vi "Prototype with Standard Deviation.vi"() -> ()   [LabVIEW 2012]
doc: "Use this template to build a standard state machine design pattern. Each state executes code and determines which state to transition to. Contrast this design pattern with the User Interface Event Handler pattern, in which code executes in response to user actions. Contrast this design pattern also with the Queued Message Handler pattern, in which each message handling code can queue zero or more new messages.\nNote: This template does not contain the most recent programming guidelines recommended by National Instruments. For a complete, project-based implementation of the Standard State Machine pattern, use the Create Project dialog box instead of this template."
uses:
  <vilib>/Math Plots/3D Math Plots/3D Bar/3D Bar Datatype/3D Bar Datatype.lvclass
  <vilib>/Math Plots/3D Math Plots/3D Bar/3D Bar Datatype/Public/Plot Helper (Vector).vi
  <vilib>/Math Plots/3D Math Plots/3D Bar/3D Bar XCtrl/3D Bar.xctl
panel:
  out "Tramp contact":bool
  out "3D Bar Graph":refnum<class "3D Plot Datatype.lvclass">[](xcontrol)
  out "Total Air Time":dbl
  out "Number of\nTotal Jumps":i32
  out "Number of Official Jumps":i32
  in  "Start Official Jumps \n(Represents Current State)":bool
  out "Final Jump Times":dbl[](array[numeric])
  out "Trampoline Time":dbl[](array[numeric])
  out "Air Time":dbl[](array[numeric])
  in  "Stop":bool
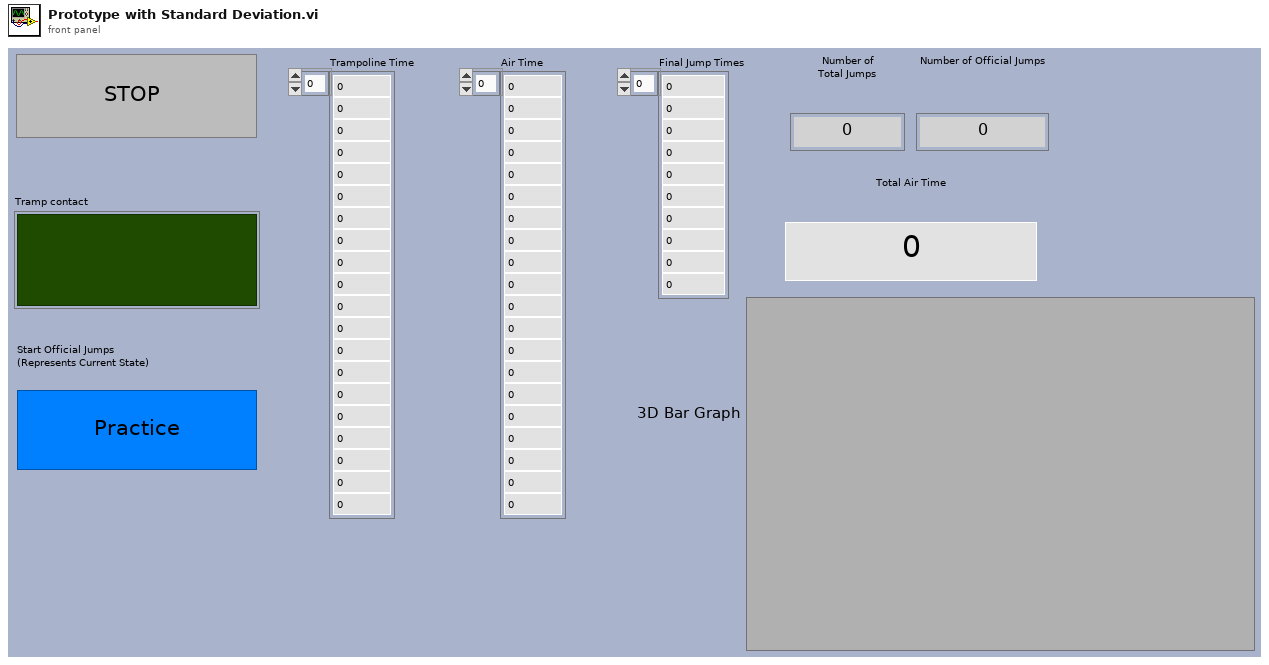
[diagram p1: front panel]
types:
  T1 = cluster{"On Trampoline":bool, "Timestamp":timestamp}
  T2 = cluster{"Start Time":dbl, "Air Time Array ":dbl[], "Tramp Time Array":dbl[], "Number of Jumps  ":i32, "Tramp switch":bool, "Final Time Array":dbl[], "Number of Final Jumps":i32}
  T3 = enum16{"Initialize", "acquire", "analyze", "display", "Stop"}
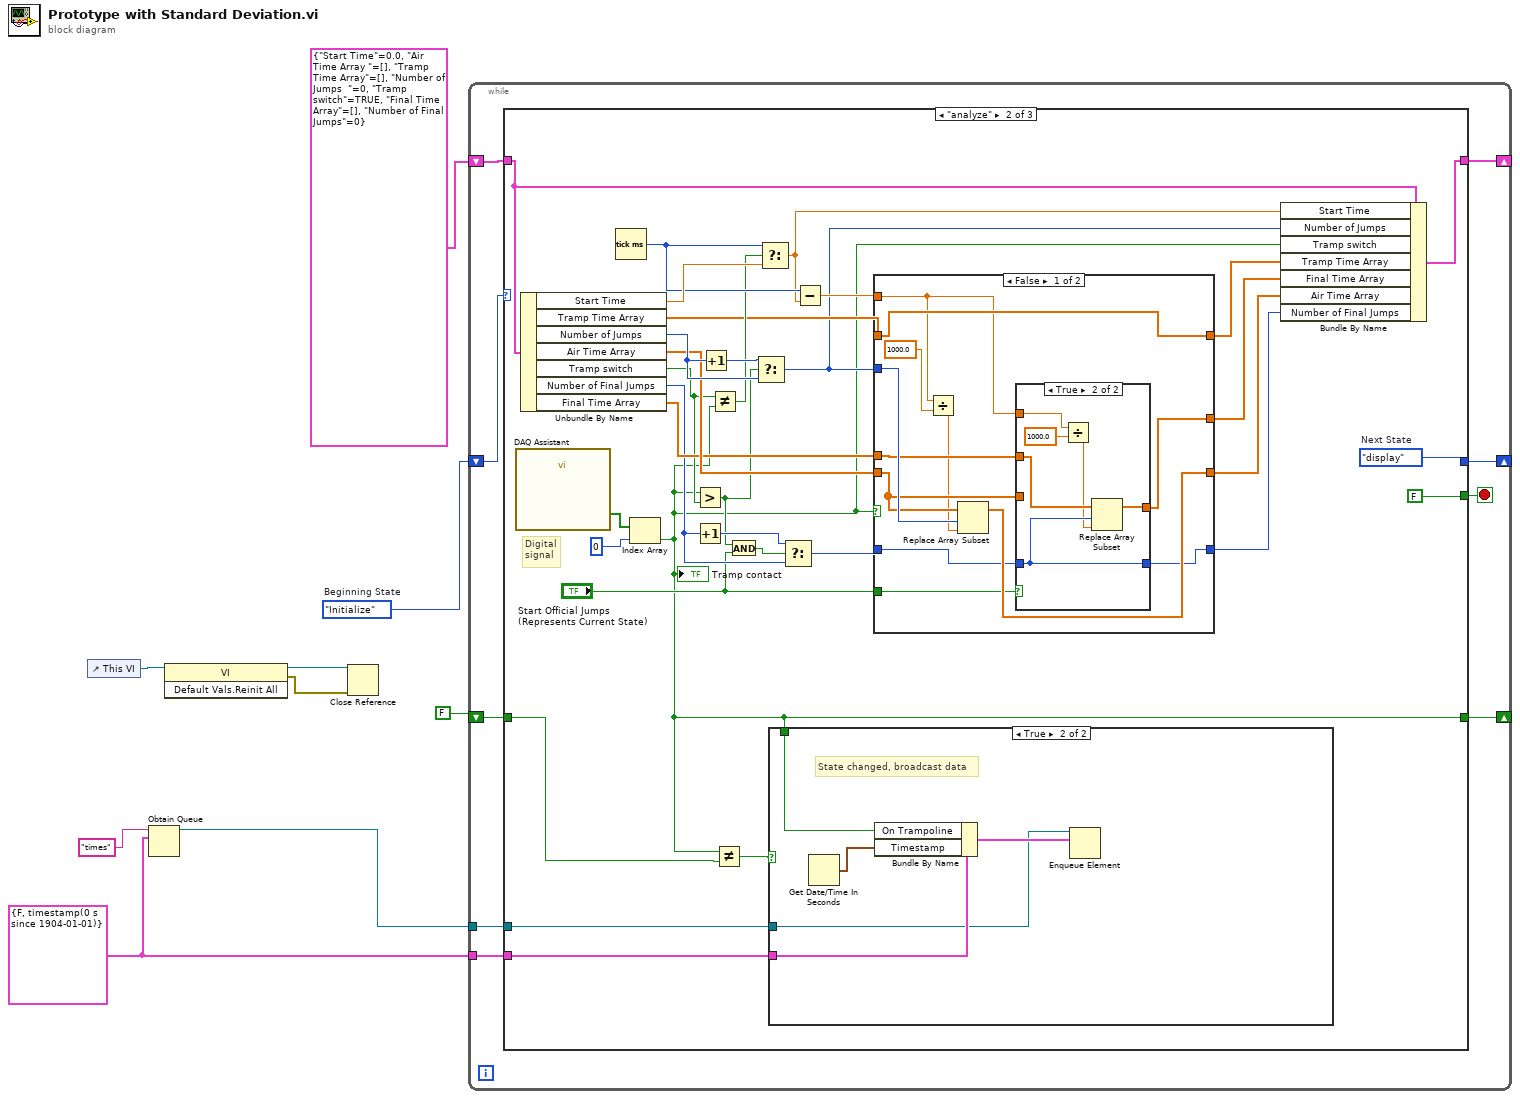
[diagram p0: block diagram]
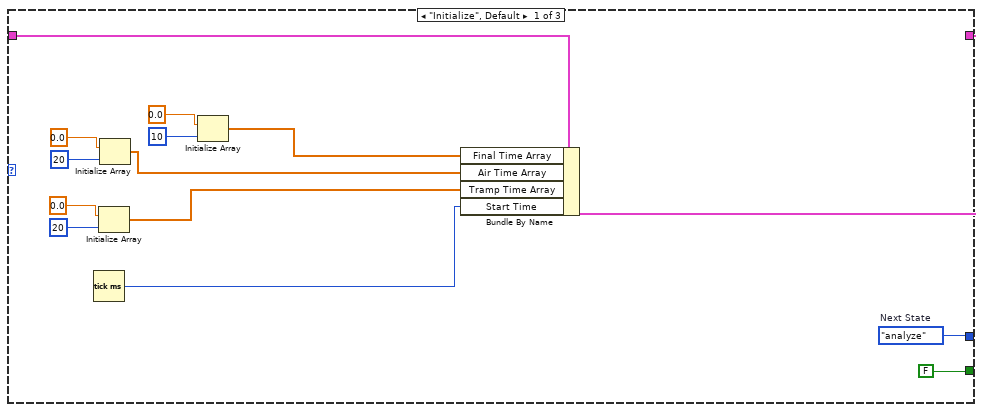
[diagram p2: hidden frame]
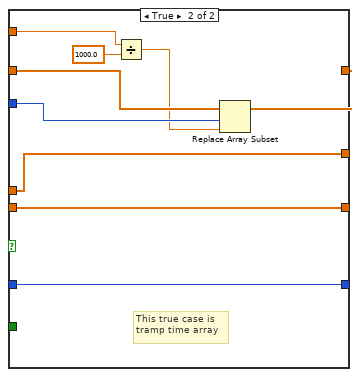
[diagram p5: hidden frame]
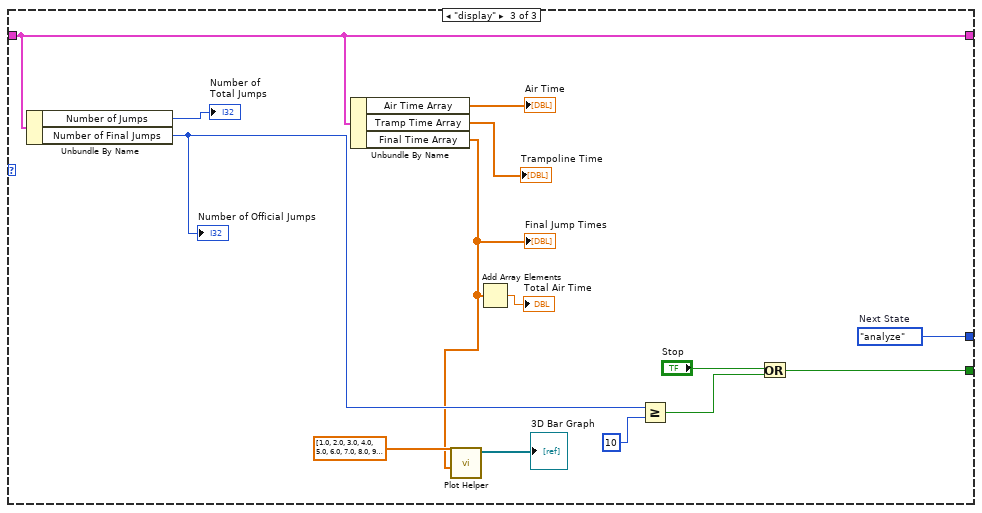
[diagram p6: hidden frame]
diagram:
  w2 = T1 {"On Trampoline"=FALSE, "Timestamp"=timestamp(0 s since 1904-01-01)}
  w9 = T3."Initialize"  # Beginning State
  n1 = control-ref of="This VI"() -> (w7:refnum<vi>)
  n2 = Obtain Queue(name (unnamed)="times", element data type=w2) -> (queue out=w1:refnum<queue>)  [unwired: 3 in, 2 out]
  n3 = invoke class="VI" method="Default Vals.Reinit All"(reference=w7) -> (reference out=w6:refnum<vi>, error out=w5:errorcluster)  [unwired: 2 in, 1 out]
  n4 = Close Reference(reference=w6, error in (no error)=w5) -> ()  [unwired: 1 out]
  n5 = while {
    shift-right: [w15] -> _
    shift-left: w9 -> [w18]
    shift-right: [w16] -> _
    shift-left: T2 {"Start Time"=0.0, "Air Time Array "=[], "Tramp Time Array"=[], "Number of Jumps  "=0, "Tramp switch"=TRUE, "Final Time Array"=[], "Number of Final Jumps"=0} -> [w17]
    shift-right: [w13] -> _
    shift-left: FALSE -> [w12]
    tunnel: w2 -> [w11]
    tunnel: w1 -> [w10]
    stop <- w14 stop-if-true
    n6 = case shown="\"analyze\"" w18 {
      tunnel: [w32 w65 w113] -> w15
      tunnel: w17 -> [w31 w62 w108]
      tunnel: [w23 w63 w108] -> w16
      tunnel: [FALSE FALSE w111] -> w14
      tunnel: [_ w35 _] -> w13
      tunnel: w12 -> [_ w37 _]
      tunnel: w11 -> [_ w34 _]
      tunnel: w10 -> [_ w33 _]
      frame "Initialize", Default {
        w32 = T3."analyze"  # Next State
        n7 = Tick Count (ms)() -> (millisecond timer value=w19:u32)
        n8 = Initialize Array "Initialize Array"(0.0 ("element"), 20 ("dimension size")) -> (w24:dbl[])
        n9 = Initialize Array(0.0 ("element"), 20 ("dimension size")) -> (w27:dbl[])
        n10 = Initialize Array(0.0 ("element"), 10 ("dimension size")) -> (w20:dbl[])
        n11 = Bundle By Name(cluster=w31, "Final Time Array"=w20, "Air Time Array"=w27, "Tramp Time Array"=w24, "Start Time"=w19) -> (w23:T2)
      }
      frame "analyze" {
        w65 = T3."display"  # Next State
        # "Digital\nsignal"
        n12 = call "DAQ Assistant"() -> ("data"=w40:bool[])  [unwired: 17 in, 2 out]
        n13 = Unbundle By Name(w62) -> ("Start Time"=w59:dbl, "Tramp Time Array"=w55:dbl[], "Number of Jumps"=w60:i32, "Air Time Array"=w56:dbl[], "Tramp switch"=w38:bool, "Number of Final Jumps"=w50:i32, "Final Time Array"=w53:dbl[])
        n14 = Tick Count (ms)() -> (millisecond timer value=w58:u32)
        n15 = Index Array(array=w40, index=0) -> (element=w35:bool)
        "Tramp contact" <- w35
        n16 = Greater?(x=w35, y=w38) -> (0:w48:bool)
        n17 = Increment(x=w50) -> (x+1=w51:i32)
        n18 = Increment(x=w60) -> (x+1=w61:i32)
        n19 = Not Equal?(x=w38, y=w35) -> (x != y?=w57:bool)
        n20 = Not Equal?(x=w35, y=w37) -> (x != y?=w36:bool)
        n21 = And(x=w48, y="Start Official Jumps \n(Represents Current State)") -> (x .and. y?=w47:bool)
        n22 = Select(t=w61, s=w48, f=w60) -> (s? t:f=w44:i32)
        n23 = Select(t=w58, s=w57, f=w59) -> (s? t:f=w43:dbl)
        n24 = case shown="True" w36 {
          tunnel: w35 -> [_ w69]
          tunnel: w34 -> [_ w68]
          tunnel: w33 -> [_ w66]
          frame False {
          }
          frame True {
            # "State changed, broadcast data"
            n25 = Get Date/Time In Seconds() -> (seconds since 1Jan1904=w70:timestamp)
            n26 = Bundle By Name(cluster=w68, "On Trampoline"=w69, "Timestamp"=w70) -> (w67:T1)
            n27 = Enqueue Element(queue=w66, element=w67) -> ()  [unwired: 2 in, 3 out]
          }
        }
        n28 = Select(t=w51, s=w47, f=w50) -> (s? t:f=w49:i32)
        n29 = Subtract(x=w58, y=w43) -> (x-y=w54:dbl)
        n30 = case shown="False" w35 {
          tunnel: [w81 w99] -> w42
          tunnel: [w82 w96] -> w45
          tunnel: w56 -> [w79 w96]
          tunnel: w55 -> [w81 w98]
          tunnel: w44 -> [w80 w97]
          tunnel: w54 -> [w71 w92]
          tunnel: w53 -> [w77 w95]
          tunnel: [w78 w95] -> w46
          tunnel: w49 -> [w76 w94]
          tunnel: [w75 w94] -> w52
          tunnel: "Start Official Jumps \n(Represents Current State)" -> [w74 _]
          frame False {
            n31 = Divide(x=w71, y=1000.0) -> (x/y=w72:dbl)
            n32 = Replace Array Subset(array=w79, new element=w72, index=w80) -> (w82:dbl[])
            n33 = case shown="True" w74 {
              tunnel: w71 -> [_ w85]
              tunnel: w79 -> [_ _]
              tunnel: [w84 w89] -> w78
              tunnel: w77 -> [w84 w90]
              tunnel: w76 -> [w83 w88]
              tunnel: [w83 w88] -> w75
              frame False {
              }
              frame True {
                n34 = Divide(x=w85, y=1000.0) -> (x/y=w86:dbl)
                n35 = Replace Array Subset(array=w90, new element=w86, index=w88) -> (w89:dbl[])
              }
            }
          }
          frame True {
            # "This true case is tramp time array"
            n36 = Divide(x=w92, y=1000.0) -> (x/y=w91:dbl)
            n37 = Replace Array Subset "Replace Array Subset"(array=w98, new element=w91, index=w97) -> (w99:dbl[])
          }
        }
        n38 = Bundle By Name(cluster=w62, "Start Time"=w43, "Number of Jumps"=w44, "Tramp switch"=w35, "Tramp Time Array"=w42, "Final Time Array"=w46, "Air Time Array"=w45, "Number of Final Jumps"=w52) -> (w63:T2)
      }
      frame "display" {
        w113 = T3."analyze"  # Next State
        n39 = Unbundle By Name(w108) -> ("Number of Jumps"=→"Number of\nTotal Jumps":i32, "Number of Final Jumps"=w105:i32)
        "Number of Official Jumps" <- w105
        n40 = Unbundle By Name(w108) -> ("Air Time Array"=→"Air Time":dbl[], "Tramp Time Array"=→"Trampoline Time":dbl[], "Final Time Array"=w100:dbl[])
        "Final Jump Times" <- w100
        n41 = call-poly <vilib>:"Plot Helper.vi"("z vector"=w100, "y vector"=sgl[] [1.0, 2.0, 3.0, 4.0, 5.0, 6.0, 7.0, 8.0, 9.0, 10.0]) -> ("3D Plot lvclass Array out"=→"3D Bar Graph":refnum<class "3D Plot Datatype.lvclass">[])  [unwired: 1 in, 8 out]
        n42 = Add Array Elements(numeric array=w100) -> (sum=→"Total Air Time":dbl)
        n43 = Greater Or Equal?(x=w105, y=10) -> (x >= y?=w110:bool)
        n44 = Or(x="Stop", y=w110) -> (x .or. y?=w111:bool)
      }
    }
  }
